vi "LJstreamM apply formula to array.vi"(0 "Index":i32, 1 "Input Values":dbl[][](array[numeric]) format="%.2f", 2 "Variables Input":string[](array[string])=["v1", "v2", "v3", "v4"], 3 "formula":string, 4 "error in (no error)":errorcluster) -> (5 "Output Values":dbl[](array[numeric]) format="%.2f", 6 "error out":errorcluster)   [LabVIEW 2025]
doc: "Similar to the Formula Node function, but with variables that can be entered on the front panel."
uses:
  <vilib>/gmath/NI_Gmath.lvlib
panel:
  in  "Variables Output":string[](array[string])=["y"]
  # "Input = v\nOutput = y"
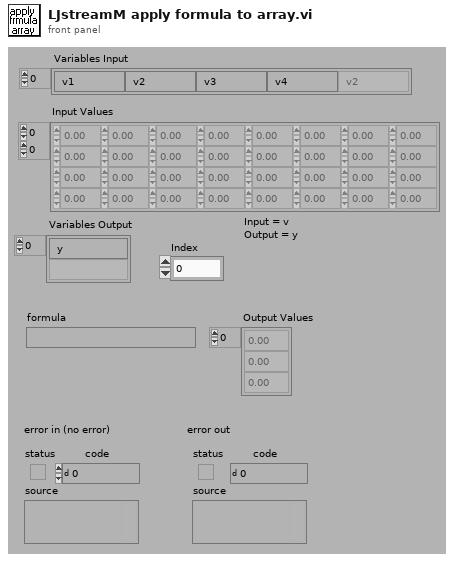
[diagram p1: front panel]
types:
  T1 = cluster{"Y Values":dbl[][], "Tables":i32[][][], "Variables input decode":i32[], "Variables output decode":i32[]}
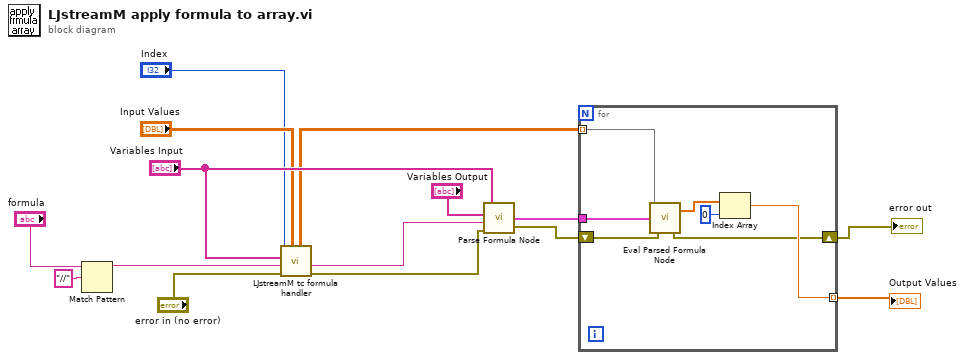
[diagram p0: block diagram]
diagram:
  n1 = Match Pattern(string="formula", regular expression="//") -> (before substring=w3:string)  [unwired: 1 in, 3 out]
  n2 = call "LJstreamM tc formula handler.vi"("Input Values In"="Input Values", "error in (no error)"="error in (no error)", "formula"=w3, "Variables Input"="Variables Input", "Index"="Index") -> ("error out"=w1:errorcluster, "formula out"=w7:string, "Input Values Out"=w6:dbl[][])  [unwired: 2 in]
  n3 = call <vilib>:"Parse Formula Node.vi"("error in (no error)"=w1, "formula"=w7, "Variables Output"="Variables Output", "Variables Input"="Variables Input") -> ("error out"=w14:errorcluster, "Parsed Formula Node"=w13:T1)
  n4 = for {
    tunnel: w6 -> [w16] mode=indexing
    tunnel: w13 -> [w22]
    tunnel: [w19] -> w12 mode=indexing
    shift-right: [w17] -> w15
    shift-left: w14 -> [w18]
    n5 = call <vilib>:"Eval Parsed Formula Node.vi"("error in (no error)"=w18, "Parsed Formula Node"=w22, "Input Values"=w16) -> ("error out"=w17:errorcluster, "Output Values"=w21:dbl[])
    n6 = Index Array(array=w21, index=0 ("Index")) -> (element=w19:dbl)
  }
  "Output Values" <- w12
  "error out" <- w15
